vi "QueueWarnings.vi"(8 "Warning":string, 10 "Text.Text in":string, 11 "Masks":string) -> (3 "Text.Text out":string)   [LabVIEW 2020]
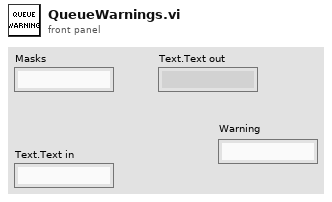
[diagram p1: front panel]
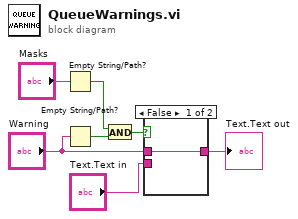
[diagram p0: block diagram]
diagram:
  n1 = Empty String/Path?(string/path="Masks") -> (empty?=w5:bool)
  n2 = Empty String/Path?(string/path="Warning") -> (empty?=w2:bool)
  n3 = And(x=w5, y=w2) -> (x .and. y?=w3:bool)
  n4 = case shown="False" w3 {
    tunnel: [w8 w9] -> w7
    tunnel: "Text.Text in" -> [_ w9]
    tunnel: "Warning" -> [w8 _]
    frame False {
    }
    frame True {
    }
  }
  "Text.Text out" <- w7
